vi "ForceRedraw.vi"(8 "error in":errorcluster, 11 "Waveform Chart ref":refnum<vi>) -> (0 "error out":errorcluster)   [LabVIEW 2016]
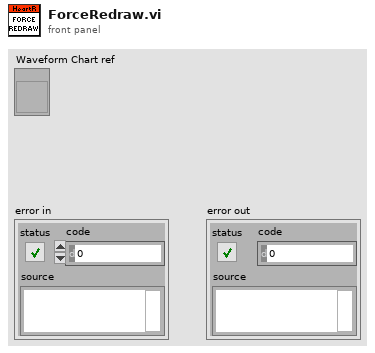
[diagram p1: front panel]
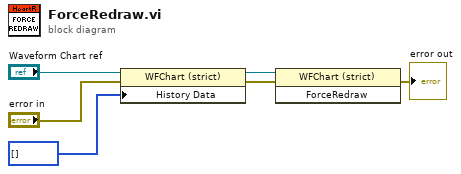
[diagram p0: block diagram]
diagram:
  n1 = property on="Property Node" class="WFChart (strict)"(reference="Waveform Chart ref", error in="error in", "History Data"=i32[] []) -> (reference out=w2:refnum<vi>, error out=w6:errorcluster)
  n2 = invoke on="Invoke Node" class="WFChart (strict)" method="ForceRedraw"(reference=w2, error in=w6) -> (error out=→"error out":errorcluster)  [unwired: 1 in, 2 out]
